vi "Tank 2 Blower Interlock Configuration.vi"(8 "error in (no error)":errorcluster, 11 "cRIO-CO2 in":refnum<class "cRIO-CO2.lvclass">) -> (0 "error out":errorcluster, 2 "Interlock Chain":refnum<class "Interlock Chain.lvclass">, 3 "cRIO-CO2 out":refnum<class "cRIO-CO2.lvclass">)   [LabVIEW 2015, in "cRIO-Carbondioxide.lvlib" / "cRIO-CO2.lvlib" / "cRIO-CO2.lvclass"]
uses:
  cRIO-CO2.lvclass
  Interlocks/Interlock Chain/Interlock Chain.lvclass
  Interlocks/Interlock/Interlock.lvclass
  Interlocks/Interlock Bool/Interlock Bool.lvclass
  Interlocks/Interlock Bool/Interlock Bool.lvclass/Interlock Bool.ctl
  Interlocks/Interlock Chain/Interlock Chain.lvclass/Interlock Chain.ctl
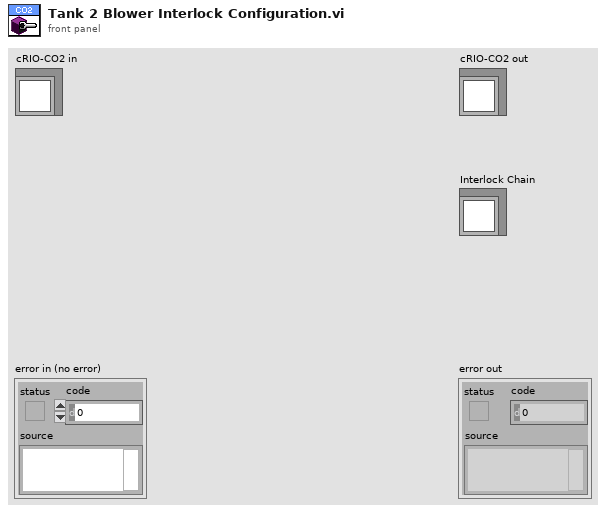
[diagram p1: front panel]
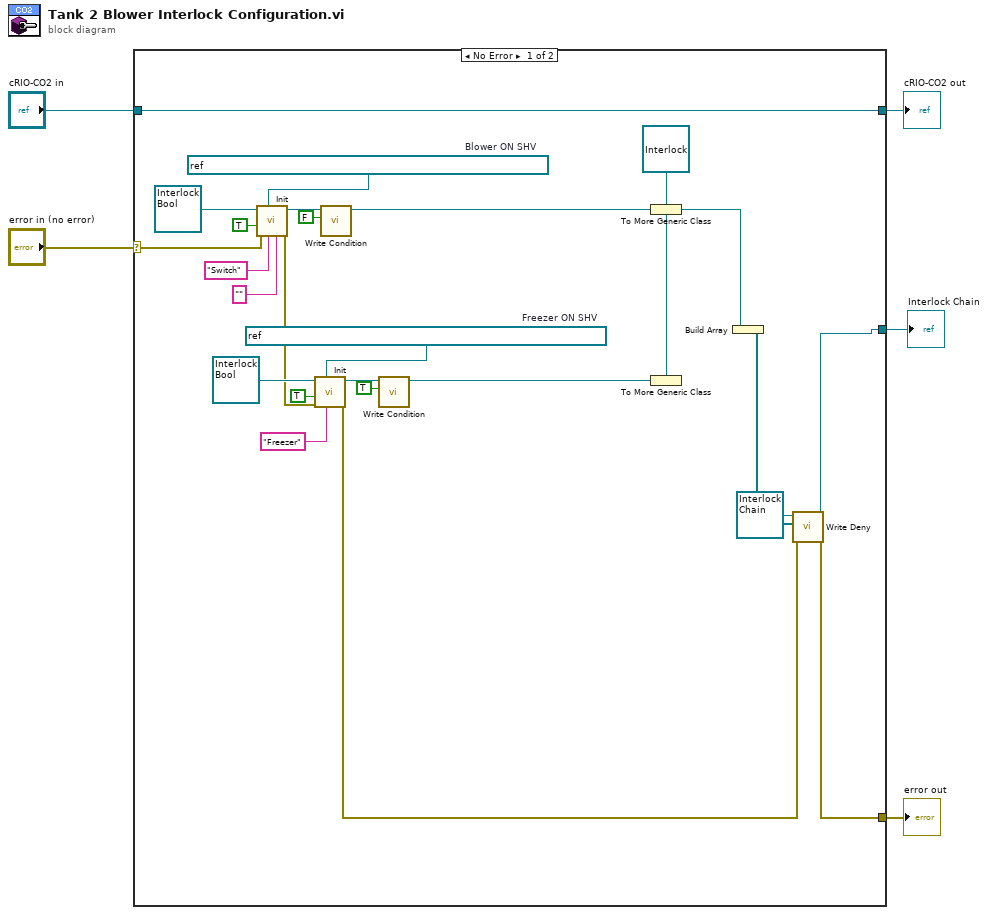
[diagram p0: block diagram]
diagram:
  n1 = case shown="No Error" "error in (no error)" {
    selector: "error in (no error)" -> [w16 w32]
    tunnel: [w10 w32] -> w4
    tunnel: [w30 w31] -> w2
    tunnel: "cRIO-CO2 in" -> [w30 w31]
    tunnel: [w8 _] -> w1
    frame No Error {
      w19 = refnum<k21> "ni.var.psp://10.2.0.20/AMS Gas SHV/Freezers/Freezer Tank 2"  # Freezer ON SHV
      w27 = refnum<k21> "ni.var.psp://10.2.0.20/AMS Gas SHV/Blowers/Tank Blower 2"  # Blower ON SHV
      w13 = refnum<class "Interlock.lvclass"> refnum ("Interlock.lvclass")
      n2 = call-dynamic "Init.vi"("Interlock message (\" -> Interlock!\")"="" ("Interlock message (\" -> Interlock!\")"), "Name (SHV Name if empty)"="Switch", "SHV"=w27, "error in (no error)"=w16, "Stop Self on IL? (T)"=TRUE, "Interlock in"=refnum<class "Interlock Bool.lvclass"> refnum ("Interlock Bool.lvclass")) -> ("error out"=w15:errorcluster, "Interlock out"=w28:refnum<class "Interlock Bool.lvclass">)  [unwired: 4 in]
      n3 = call-dynamic "Init.vi"("Name (SHV Name if empty)"="Freezer", "SHV"=w19, "error in (no error)"=w15, "Stop Self on IL? (T)"=TRUE, "Interlock in"=refnum<class "Interlock Bool.lvclass"> refnum ("Interlock Bool.lvclass")) -> ("error out"=w11:errorcluster, "Interlock out"=w18:refnum<class "Interlock Bool.lvclass">)  [unwired: 5 in]
      n4 = call "Write Condition.vi"("Interlock Condition"=FALSE, "Interlock Bool in"=w28) -> ("Interlock Bool out"=w24:refnum<class "Interlock Bool.lvclass">)  [unwired: 8 in, 1 out]
      n5 = call "Write Condition.vi"("Interlock Condition"=TRUE, "Interlock Bool in"=w18) -> ("Interlock Bool out"=w14:refnum<class "Interlock Bool.lvclass">)  [unwired: 8 in, 1 out]
      n6 = To More Generic Class(target class=w13, reference=w24) -> (generic class reference=w23:refnum<class "Interlock.lvclass">)
      n7 = To More Generic Class(target class=w13, reference=w14) -> ()  [unwired: 1 out]
      n8 = Build Array(w23) -> (w9:refnum<class "Interlock.lvclass">[])
      n9 = call "Write Deny.vi"("error in (no error)"=w11, "Deny"=w9, "Interlock Chain in"=refnum<class "Interlock Chain.lvclass"> refnum) -> ("error out"=w10:errorcluster, "Interlock Chain out"=w8:refnum<class "Interlock Chain.lvclass">)  [unwired: 7 in]
    }
    frame Error {
    }
  }
  "error out" <- w4
  "cRIO-CO2 out" <- w2
  "Interlock Chain" <- w1
